vi "setViTitle.vi"(8 "error in (no error)":errorcluster, 10 "Path":path, 11 "ScriptEditorV2 in":refnum<class "ScriptEditorV2.lvclass">) -> (0 "error out":errorcluster, 3 "ScriptEditorV2 out":refnum<class "ScriptEditorV2.lvclass">)   [LabVIEW 2011, in "Views.lvlib" / "ScriptEditor.lvlib" / "ScriptEditorV2.lvclass"]
uses:
  ScriptEditorV2.lvclass
  ScriptEditorV2.lvclass/ScriptEditorV2.ctl
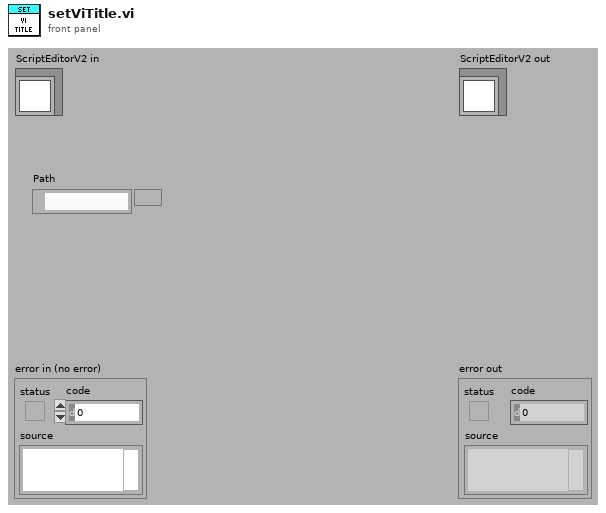
[diagram p1: front panel]
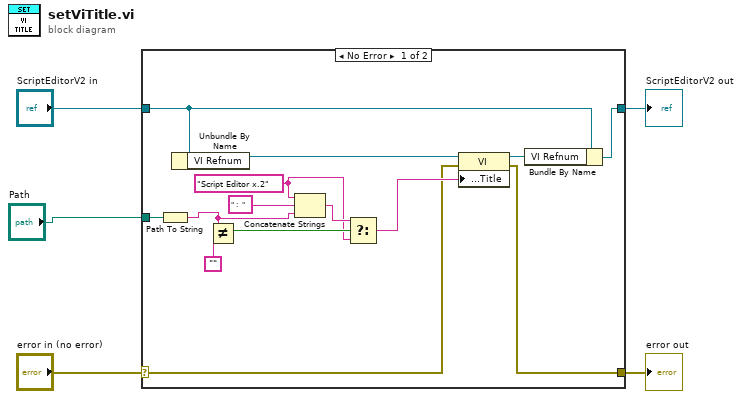
[diagram p0: block diagram]
diagram:
  n1 = case shown="No Error" "error in (no error)" {
    selector: "error in (no error)" -> [w12 w21]
    tunnel: [w11 w21] -> w4
    tunnel: [w8 w20] -> w2
    tunnel: "ScriptEditorV2 in" -> [w9 w20]
    tunnel: "Path" -> [w7 _]
    frame No Error {
      w14 = "Script Editor x.2"
      n2 = Path To String(path=w7) -> (string=w6:string)
      n3 = Unbundle By Name(w9) -> ("VI Refnum"=w19:refnum<vi>)
      n4 = Not Equal?(x=w6, y="") -> (x != y?=w17:bool)
      n5 = Concatenate Strings(w14, " :  ", w6) -> (w16:string)
      n6 = Select(t=w16, s=w17, f=w14) -> (s? t:f=w13:string)
      n7 = property class="VI"(reference=w19, error in=w12, "Front Panel.Title"=w13) -> (reference out=w10:refnum<vi>, error out=w11:errorcluster)
      n8 = Bundle By Name(cluster=w9, "VI Refnum"=w10) -> (w8:refnum<class "ScriptEditorV2.lvclass">)
    }
    frame Error {
    }
  }
  "error out" <- w4
  "ScriptEditorV2 out" <- w2
